vi "loadNodes.vi"(8 "error in (no error)":errorcluster, 11 "xceRootNode in":refnum<class "xceRootNode.lvclass">) -> (0 "error out":errorcluster, 1 "cancelled":bool, 3 "xceRootNode out":refnum<class "xceRootNode.lvclass">)   [LabVIEW 2014, in "xceRootNode.lvclass"]
doc: "Starts the loading process for an existing configuration file."
uses:
  xceRootNode.lvclass
  XML Parser/lineCounter_action.ctl
  xceRootNode.lvclass/xceRootNode.ctl
  xceDataNode/xceDataNode.lvclass
  xceNode/xceNode.lvclass
  XML Parser/XML Parser.lvclass
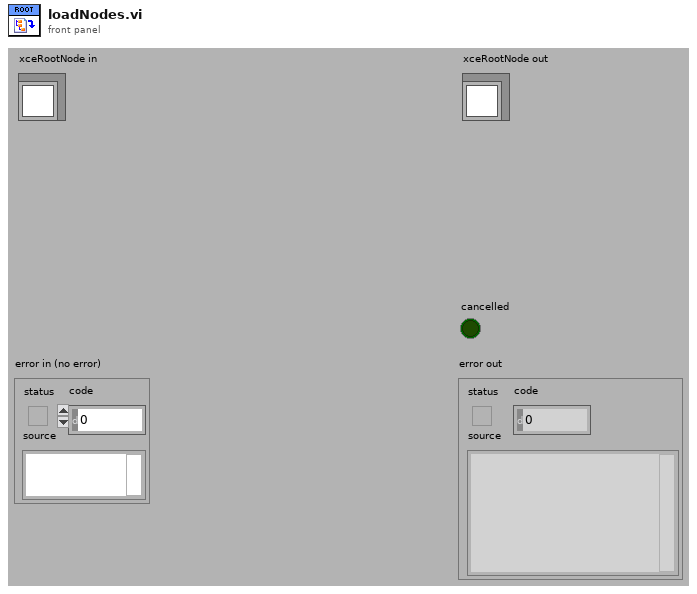
[diagram p1: front panel]
types:
  T1 = typedef "XML Parser.lvclass/lineCounter_action.ctl" = enum16{"Init", "Reset", "Increment", "Get Current Line"}
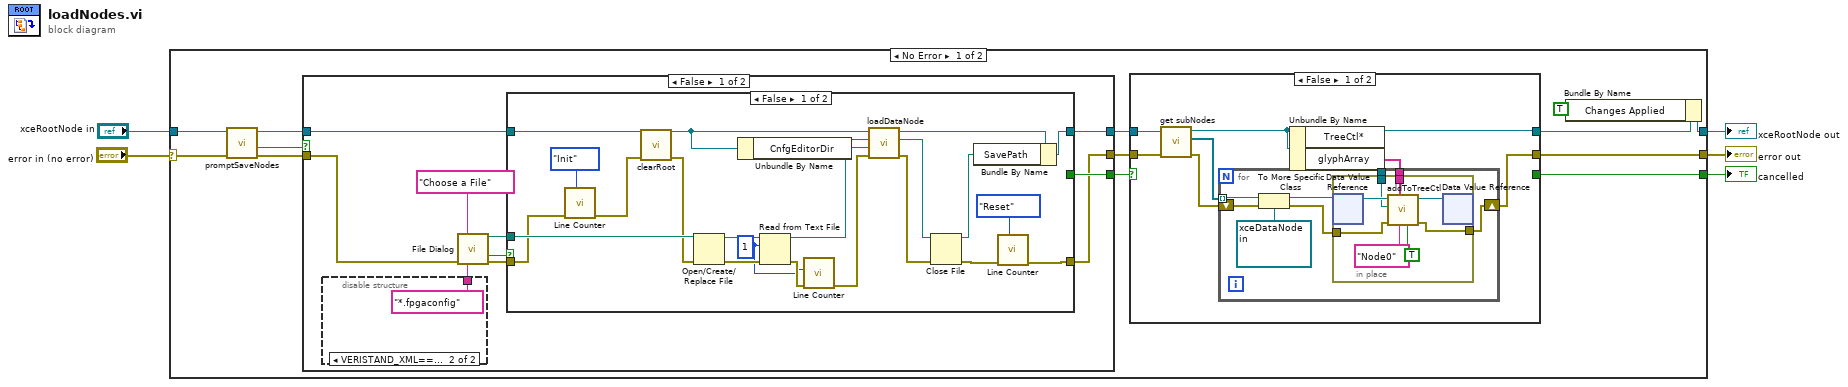
[diagram p0: block diagram]
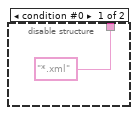
[diagram p3: hidden frame]
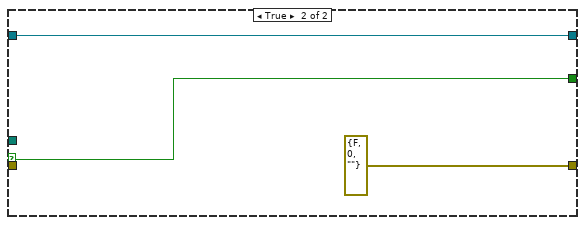
[diagram p4: hidden frame]
diagram:
  n1 = case shown="No Error" "error in (no error)" {
    selector: "error in (no error)" -> [w16 w87]
    tunnel: [w10 w87] -> w4
    tunnel: [w6 w86] -> w2
    tunnel: "xceRootNode in" -> [w18 w86]
    tunnel: [w9 _] -> w1
    frame No Error {
      n2 = call "promptSaveNodes.vi"("error in (no error)"=w16, "xceRootNode in"=w18) -> ("error out"=w15:errorcluster, "cancelled"=w14:bool, "xceRootNode out"=w17:refnum<class "xceRootNode.lvclass">)  [unwired: 7 in]
      n3 = case shown="False" w14 {
        selector: w14 -> [_ w84]
        tunnel: [w52 w84] -> w13
        tunnel: [w49 w85] -> w12
        tunnel: [w48 w83] -> w11
        tunnel: w17 -> [w46 w85]
        tunnel: w15 -> [w47 w83]
        frame False {
          n4 = disable-structure shown="VERISTAND_XML==True" {
            disable-tunnel: ["*.xml" ("pattern (all files)") "*.fpgaconfig" ("pattern (all files)")] -> w54
            frame condition #0 {
            }
            frame condition #1 (active) {
            }
          }
          n5 = call "File Dialog"("prompt"="Choose a File", "error in"=w47, "pattern (all files)"=w54) -> ("selected path"=w50:path, "cancelled"=w53:bool, "error out"=w51:errorcluster)  [unwired: 9 in, 1 out]
          n6 = case shown="False" w53 {
            selector: w53 -> [_ w82]
            tunnel: [_ w82] -> w52
            tunnel: w51 -> [w66 _]
            tunnel: w50 -> [w79 _]
            tunnel: w46 -> [w72 w81]
            tunnel: [w59 errorcluster {"status"=FALSE, "code"=0, "source"=""} ("error out")] -> w48
            tunnel: [w67 w81] -> w49
            frame False {
              w61 = 1 ("count")
              n7 = call "Line Counter.vi"("Action (Increment)"=lineCounter_action."Init" ("Action"), "error in (no error)"=w66) -> ("error out"=w64:errorcluster)  [unwired: 8 in, 1 out]
              n8 = call "clearRoot.vi"("error in (no error)"=w64, "xceRootNode in"=w72) -> ("error out"=w70:errorcluster, "xceRootNode out"=w71:refnum<class "xceRootNode.lvclass">)  [unwired: 8 in]
              n9 = Open/Create/Replace File(file path (use dialog)=w79, error in=w70) -> (refnum out=w77:refnum<file>, error out=w78:errorcluster)  [unwired: 4 in, 1 out]
              n10 = Unbundle By Name(w71) -> ("CnfgEditorDir"=w75:path)
              n11 = Read from Text File(file (use dialog)=w77, count=w61, error in=w78) -> (refnum out=w76:refnum<file>, error out=w63:errorcluster)  [unwired: 1 in, 2 out]
              n12 = call "Line Counter.vi"("error in (no error)"=w63, "# of lines to increment (1)"=w61) -> ("error out"=w62:errorcluster)  [unwired: 8 in, 1 out]
              n13 = call "loadDataNode.vi"("error in (no error)"=w62, "CnfgEditorDir"=w75, "XML Refnum in"=w76, "xceDataNode in"=w71) -> ("error out"=w74:errorcluster, "XML Refnum out"=w73:refnum<file>, "xceDataNode out"=w68:refnum<class "xceRootNode.lvclass">)  [unwired: 5 in]
              n14 = Close File(refnum=w73, error in=w74) -> (path=w69:path, error out=w60:errorcluster)
              n15 = Bundle By Name(cluster=w68, "SavePath"=w69) -> (w67:refnum<class "xceRootNode.lvclass">)
              n16 = call "Line Counter.vi"("Action (Increment)"=lineCounter_action."Reset", "error in (no error)"=w60) -> ("error out"=w59:errorcluster)  [unwired: 8 in, 1 out]
            }
            frame True {
            }
          }
        }
        frame True {
        }
      }
      n17 = case shown="False" w13 {
        selector: w13 -> [_ w43]
        tunnel: w12 -> [w26 w45]
        tunnel: [w22 w45] -> w8
        tunnel: w11 -> [w25 w44]
        tunnel: [w20 w44] -> w10
        tunnel: [_ w43] -> w9
        frame False {
          n18 = call "get subNodes.vi"("error in (no error)"=w25, "xceNode in"=w26) -> ("error out"=w24:errorcluster, "subNodes[]*"=w23:refnum<data-value>[], "xceNode out"=w22:refnum<class "xceRootNode.lvclass">)  [unwired: 7 in]
          n19 = Unbundle By Name(w22) -> ("TreeCtl*"=w21:refnum<vi>, "glyphArray"=w19:string[])
          n20 = for {
            tunnel: w23 -> [w32] mode=indexing
            tunnel: w21 -> [w30]
            shift-right: [w28] -> w20
            shift-left: w24 -> [w34]
            tunnel: w19 -> [w27]
            n21 = To More Specific Class(target class=refnum<data-value> refnum ("data value reference"), reference=w32, error in=w34) -> (specific class reference=w31:refnum<data-value>, error out=w29:errorcluster)
            n22 = in-place {
              in-place-border: w30 -> [w40]
              in-place-border: w29 -> [w39]
              in-place-border: [w38] -> w28
              in-place-border: w27 -> [w35]
              n23 = in-place-dvr #1(w31) -> (w42:refnum<class "xceDataNode.lvclass">)  [unwired: 1 out]
              n24 = call "addToTreeCtl.vi"("AppendToEnd"=TRUE, "ParentTreeTag"="Node0", "glyphArray"=w35, "error in (no error)"=w39, "TreeCtl*"=w40, "xceDataNode in"=w42) -> ("error out"=w38:errorcluster, "xceDataNode out"=w37:refnum<class "xceDataNode.lvclass">)  [unwired: 4 in]
              n25 = in-place-dvr #1(w37) -> ()  [unwired: 2 out]
            }
          }
        }
        frame True {
        }
      }
      n26 = Bundle By Name(cluster=w8, "Changes Applied"=TRUE) -> (w6:refnum<class "xceRootNode.lvclass">)
    }
    frame Error {
    }
  }
  "error out" <- w4
  "xceRootNode out" <- w2
  "cancelled" <- w1
